vi "zigzag_demo.vi"() -> ()   [LabVIEW 2017]
panel:
  in  "回零":bool
  out "状态":string
  in  "下一步":bool
  in  "开始":bool
  in  "地址":string
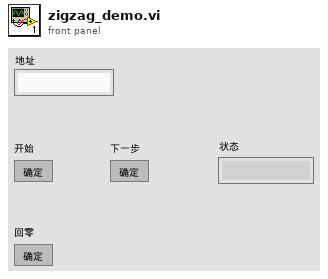
[diagram p1: front panel]
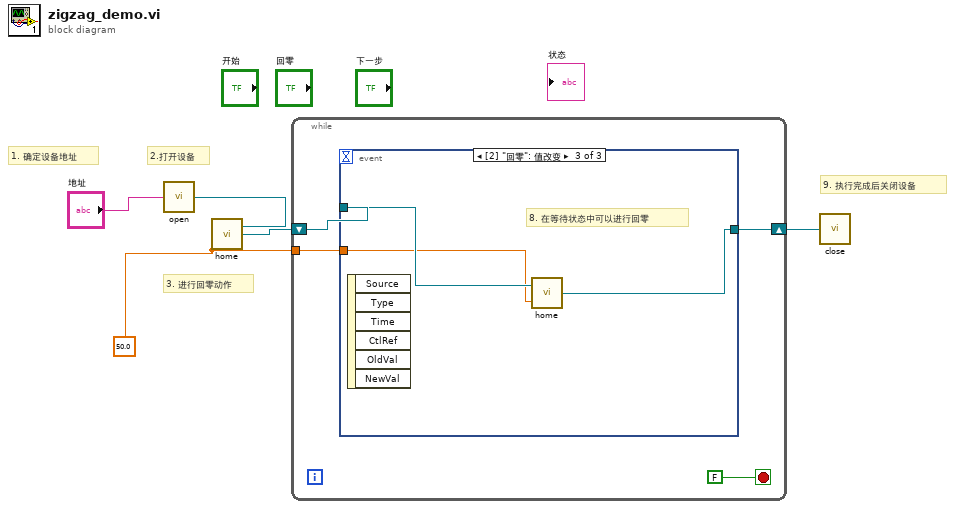
[diagram p0: block diagram]
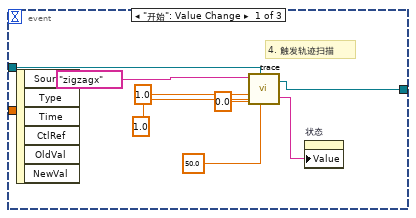
[diagram p2: hidden frame]
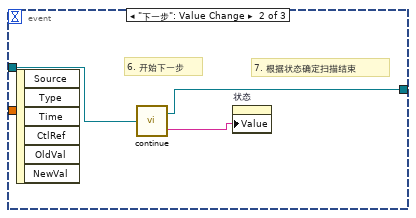
[diagram p3: hidden frame]
diagram:
  w2 = 50.0 ("速度")
  # "9. 执行完成后关闭设备"
  # "3. 进行回零动作"
  # "2.打开设备"
  # "1. 确定设备地址"
  n1 = call "open.vi"("地址"="地址") -> ("连接ID"=w5:refnum<k5>)
  n2 = call "home.vi"("速度"=w2, "连接ID"=w5) -> ("连接ID"=w3:refnum<k5>)
  n3 = while {
    tunnel: w2 -> [w8]
    shift-right: [w7] -> w1
    shift-left: w3 -> [w9]
    stop <- FALSE stop-if-true
    n4 = event shown="[2] \"回零\": 值改变" {
      selector: _ -> [_ _ _]
      dyn-events: _ -> [_ _ _]
      timeout: _ -> [_ _ _]
      tunnel: w9 -> [w17 w20 w23]
      tunnel: w8 -> [_ _ w22]
      tunnel: [w10 w18 w21] -> w7
      event "开始": Value Change {
        # "4. 触发轨迹扫描"
        n5 = event-data() -> ()  [unwired: 1 in, 6 out]
        n6 = call "trace.vi"("v"=50.0, "连接ID"=w17, "z"=0.0, "y"=1.0, "x"=1.0, "type"="zigzagx") -> ("输出状态"=w11:string, "连接ID输出"=w10:refnum<k5>)
        n7 = property on="状态" class="Str"("Value"=w11) -> ()  [unwired: 2 in, 2 out]
      }
      event "下一步": Value Change {
        # "7. 根据状态确定扫描结束"
        # "6. 开始下一步"
        n8 = event-data() -> ()  [unwired: 1 in, 6 out]
        n9 = call "continue.vi"("连接ID"=w20) -> ("连接ID"=w18:refnum<k5>, "输出状态"=w19:string)
        n10 = property on="状态" class="Str"("Value"=w19) -> ()  [unwired: 2 in, 2 out]
      }
      event "回零": Value Change {
        # "8. 在等待状态中可以进行回零"
        n11 = event-data() -> ()  [unwired: 1 in, 6 out]
        n12 = call "home.vi"("速度"=w22, "连接ID"=w23) -> ("连接ID"=w21:refnum<k5>)
      }
    }
  }
  n13 = call "close.vi"("连接ID"=w1) -> ()
